vi "judgeSecvarFormat.vi"(11 "section variable":string) -> (3 "correct format?":bool)   [LabVIEW 2010]
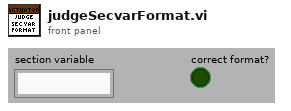
[diagram p1: front panel]
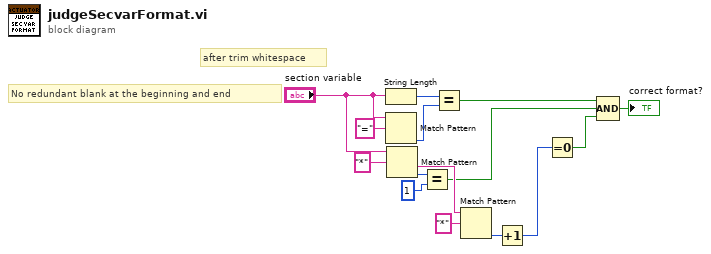
[diagram p0: block diagram]
diagram:
  # "after trim whitespace"
  # "No redundant blank at the beginning and end"
  n1 = String Length(string="section variable") -> (length=w14:i32)
  n2 = Match Pattern(string="section variable", regular expression="=") -> (offset past match=w13:i32)  [unwired: 1 in, 3 out]
  n3 = Match Pattern(string="section variable", regular expression="*") -> (after substring=w7:string, offset past match=w9:i32)  [unwired: 1 in, 2 out]
  n4 = Equal?(x=w9, y=1 ("length (rest)")) -> (x = y?=w6:bool)
  n5 = Equal?(x=w14, y=w13) -> (x = y?=w12:bool)
  n6 = Match Pattern(string=w7, regular expression="*") -> (offset past match=w5:i32)  [unwired: 1 in, 3 out]
  n7 = Increment(x=w5) -> (x+1=w3:i32)
  n8 = Equal To 0?(x=w3) -> (x = 0?=w4:bool)
  n9 = Compound Arithmetic op=AND(w12, w6, w4) -> (→"correct format?":bool)
